vi "Read Label by Line.vi"(8 "error in (no error)":errorcluster, 10 "Line":i32, 11 "gScript Interpreter in":refnum<class "gScript Interpreter.lvclass">) -> (0 "error out":errorcluster, 1 "Arguments":string[](array[string]), 2 "Label":string, 3 "gScript Interpreter out":refnum<class "gScript Interpreter.lvclass">)   [LabVIEW 2017, in "gScript Interpreter.lvclass"]
uses:
  gScript Interpreter.lvclass
  gScript Interpreter.lvclass/gScript Interpreter.ctl
  <vilib>/Utility/error.llb/Error Cluster From Error Code.vi
  <vilib>/ErrorRing/Error Ring.xnode
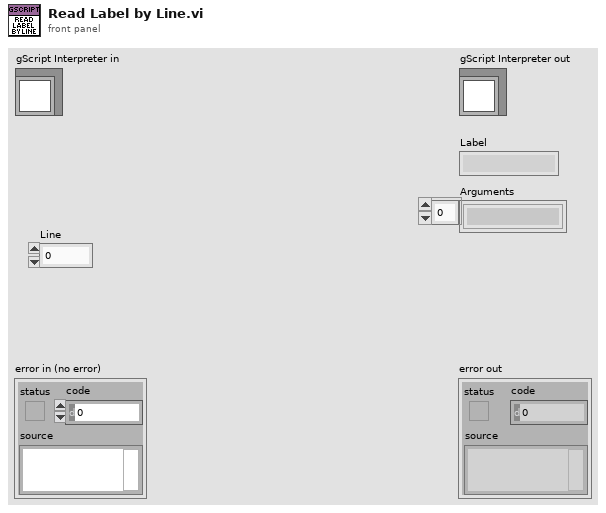
[diagram p1: front panel]
types:
  T1 = typedef "Label.ctl" = cluster{"Label":string, "Line":i32, "Arguments":string[]}
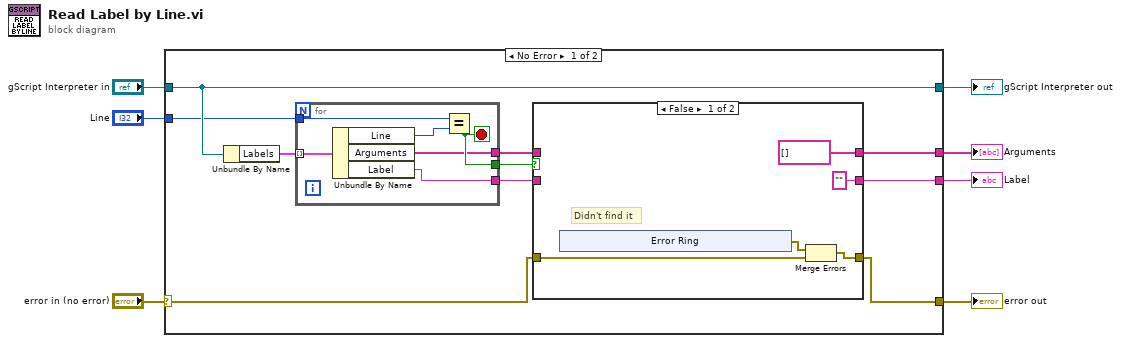
[diagram p0: block diagram]
diagram:
  n1 = case shown="No Error" "error in (no error)" {
    selector: "error in (no error)" -> [w14 w37]
    tunnel: [w13 w37] -> w6
    tunnel: [w17 w36] -> w4
    tunnel: "gScript Interpreter in" -> [w17 w36]
    tunnel: [w11 _] -> w3
    tunnel: "Line" -> [w10 _]
    tunnel: [w8 _] -> w1
    frame No Error {
      n2 = Unbundle By Name(w17) -> ("Labels"=w16:T1[])
      n3 = for {
        tunnel: w16 -> [w35] mode=indexing
        tunnel: w10 -> [w31]
        tunnel: [w34] -> w15
        tunnel: [w33] -> w12
        tunnel: [w30] -> w9
        stop <- w34 stop-if-true
        n4 = Unbundle By Name(w35) -> ("Line"=w32:i32, "Arguments"=w33:string[], "Label"=w30:string)
        n5 = Equal?(x=w31, y=w32) -> (x = y?=w34:bool)
      }
      n6 = case shown="False" w15 {
        tunnel: w14 -> [w21 w29]
        tunnel: [w20 w29] -> w13
        tunnel: w12 -> [_ w28]
        tunnel: [string[] [] ("Arguments") w28] -> w11
        tunnel: w9 -> [_ w27]
        tunnel: ["" ("Label") w27] -> w8
        frame False {
          # "Didn't find it"
          n7 = xnode "Error Ring"() -> ("error out"=w22:errorcluster)
          n8 = Merge Errors(w22, w21) -> (w20:errorcluster)
        }
        frame True {
          # "Found it"
        }
      }
    }
    frame Error {
    }
  }
  "error out" <- w6
  "gScript Interpreter out" <- w4
  "Arguments" <- w3
  "Label" <- w1
